vi "ASCII Code to String.vi"(8 "Limit to 20 Iterations?":bool=TRUE, 9 "All Characters?":bool, 10 "Array of ASCII Code":u8[](array[numeric])) -> (1 "Full String":string, 2 "Array of String Character from ASCII Code":string[](array[string]))   [LabVIEW 2016]
panel:
  out "size(s)  of array":i32
  out "length of String":i32
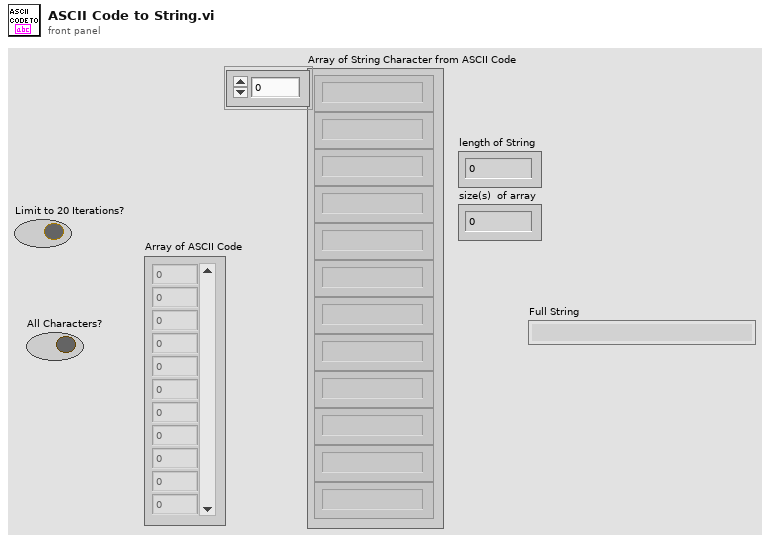
[diagram p1: front panel]
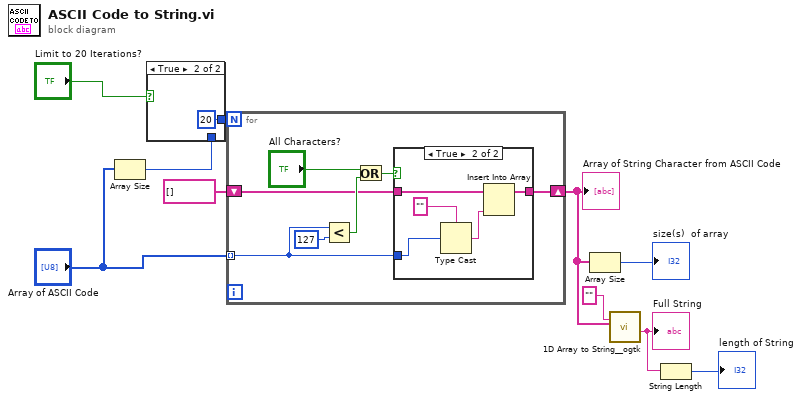
[diagram p0: block diagram]
diagram:
  n1 = Array Size(array="Array of ASCII Code") -> (size(s)=w1:i32)
  n2 = case shown="True" "Limit to 20 Iterations?" {
    tunnel: [w11 20] -> w9
    tunnel: w1 -> [w11 _]
    frame False {
    }
    frame True {
    }
  }
  n3 = for {
    N: w9 -> [_]
    tunnel: "Array of ASCII Code" -> [w19] mode=indexing
    shift-right: [w13] -> w4
    shift-left: string[] [] -> [w14]
    n4 = Less?(x=w19, y=u8 127) -> (x < y?=w17:bool)
    n5 = Or(x="All Characters?", y=w17) -> (x .or. y?=w16:bool)
    n6 = case shown="True" w16 {
      tunnel: w19 -> [_ w24]
      tunnel: [w20 w21] -> w13
      tunnel: w14 -> [w20 w23]
      frame False {
      }
      frame True {
        n7 = Type Cast(type="", x=w24) -> (*(type *) &x=w22:string)
        n8 = Insert Into Array(array=w23, new element=w22) -> (w21:string[])  [unwired: 1 in]
      }
    }
  }
  "Array of String Character from ASCII Code" <- w4
  n9 = Array Size(array=w4) -> (size(s)=→"size(s)  of array":i32)
  n10 = call <userlib>:"1D Array to String__ogtk.vi"("delimiter (Tab)"="", "Array of Strings"=w4) -> ("delimited string"=w8:string)  [unwired: 9 in]
  "Full String" <- w8
  n11 = String Length(string=w8) -> (length=→"length of String":i32)
